vi "Open Feed.vi"(8 "error in":errorcluster, 10 "create feed if necessary (F)":bool, 11 "feed folderpath":path) -> (0 "error out":errorcluster, 2 "feed created?":bool, 3 "feed folderpath out":path)   [LabVIEW 2014, in "NIPM_API.lvlib"]
doc: "Creates a new feed.\n\nIf the specified feed folderpath does not already exist, this VI will create the folder."
uses:
  NIPM_API.lvlib
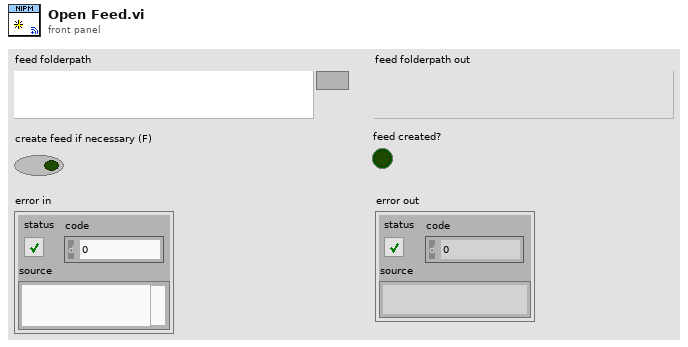
[diagram p1: front panel]
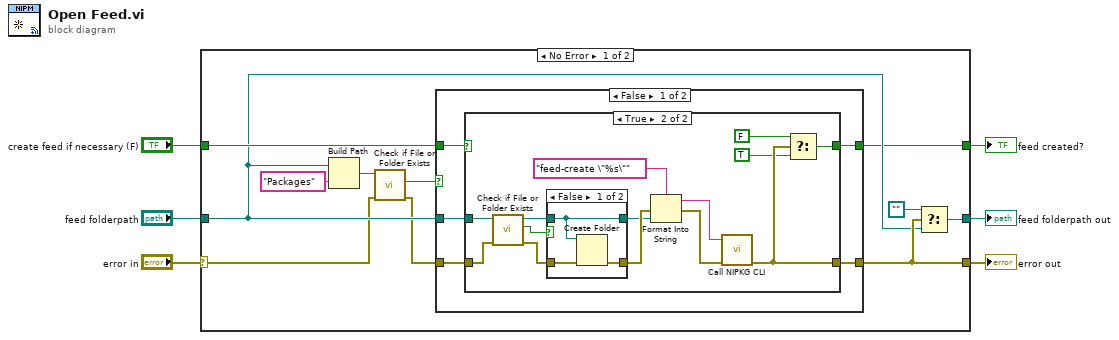
[diagram p0: block diagram]
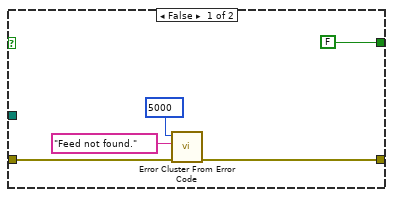
[diagram p2: hidden frame]
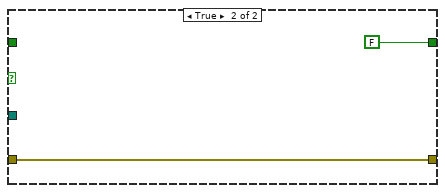
[diagram p4: hidden frame]
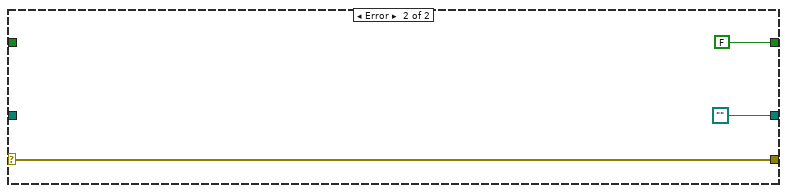
[diagram p5: hidden frame]
diagram:
  n1 = case shown="No Error" "error in" {
    selector: "error in" -> [w8 w51]
    tunnel: [w13 w51] -> w5
    tunnel: "feed folderpath" -> [w12 _]
    tunnel: [w10 path ""] -> w3
    tunnel: "create feed if necessary (F)" -> [w14 _]
    tunnel: [w9 FALSE] -> w1
    frame No Error {
      n2 = Build Path(base path=w12, name or relative path="Packages") -> (appended path=w16:path)
      n3 = call <vilib>:"Check if File or Folder Exists.vi"("error in (no error)"=w8, "path"=w16) -> ("error out"=w7:errorcluster, "file or folder exists?"=w15:bool)  [unwired: 7 in, 1 out]
      n4 = case shown="False" w15 {
        tunnel: w7 -> [w22 w48]
        tunnel: [w21 w48] -> w13
        tunnel: w12 -> [w20 _]
        tunnel: w14 -> [w19 _]
        tunnel: [w18 FALSE] -> w9
        frame False {
          n5 = case shown="True" w19 {
            tunnel: w22 -> [w25 w40]
            tunnel: [w24 w36] -> w21
            tunnel: w20 -> [_ w31]
            tunnel: [FALSE w33] -> w18
            frame False {
              n6 = call <vilib>:"Error Cluster From Error Code.vi"("error in (no error)"=w25, "error message (\"\")"="Feed not found." ("error message (\"\")"), "error code (0)"=5000) -> ("error out"=w24:errorcluster)  [unwired: 6 in]
            }
            frame True {
              n7 = call <vilib>:"Check if File or Folder Exists.vi"("error in (no error)"=w40, "path"=w31) -> ("error out"=w32:errorcluster, "file or folder exists?"=w29:bool, "dup path"=w30:path)  [unwired: 7 in]
              n8 = case shown="False" w29 {
                tunnel: [w44 w45] -> w39
                tunnel: w32 -> [w43 w45]
                tunnel: w30 -> [w42 w46]
                tunnel: [w42 w46] -> w28
                frame False {
                  n9 = Create Folder(path (use dialog)=w42, error in=w43) -> (error out=w44:errorcluster)  [unwired: 1 in, 2 out]
                }
                frame True {
                }
              }
              n10 = Format Into String(format string="feed-create \"%s\"", error in=w39, w28) -> (resulting string=w38:string, error out=w37:errorcluster)  [unwired: 1 in]
              n11 = call "Call NIPKG CLI.vi"("error in (no error)"=w37, "command"=w38) -> ("error out"=w36:errorcluster)  [unwired: 8 in, 1 out]
              n12 = Select(t=FALSE, s=w36, f=TRUE) -> (s? t:f=w33:bool)
            }
          }
        }
        frame True {
        }
      }
      n13 = Select(t=path "", s=w13, f=w12) -> (s? t:f=w10:path)
    }
    frame Error {
    }
  }
  "error out" <- w5
  "feed folderpath out" <- w3
  "feed created?" <- w1
